vi "EncodeInt32.vi"(1 "Data In":i32[](array[numeric])) -> (0 "Data Out":u8[](array[numeric]))   [LabVIEW 2014, in "navX-MXP IMU.lvlib"]
uses:
  navX-MXP IMU.lvlib
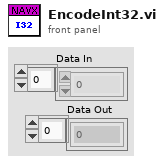
[diagram p1: front panel]
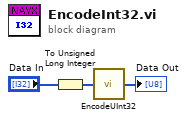
[diagram p0: block diagram]
diagram:
  n1 = To Unsigned Long Integer(number="Data In") -> (unsigned 32bit integer=w2:u32[])
  n2 = call "EncodeUInt32.vi"("Data In"=w2) -> ("Data Out"=→"Data Out":u8[])
